vi "TP_Privileges.vi"(8 "error in (no error)":errorcluster, 10 "Privilege":T1) -> (0 "error out":errorcluster)   [LabVIEW 2012]
uses:
  TP_Privileges.ctl
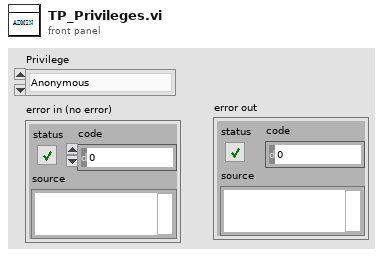
[diagram p1: front panel]
types:
  T1 = typedef "TP_Privileges.ctl" = enum16{"Anonymous", "User", "Debugger", "Developer", "Admin"}
  T2 = enum16{"Init", "GetValue", "SetValue", "Destory"}
  T3 = typedef "TP_Config.ctl" = cluster{"Info":cluster{"version":string, "date":string, "author":string, "mail":string}, "User_info":cluster{"username":string, "memery_enable":bool}, "Path":cluster{"script":string, "errlog":string}}
  T4 = typedef "TP_UI Ref.ctl" = cluster{"This VI":refnum<vi>, "String":refnum<vi>, "Test":refnum<vi>, "Quit":refnum<vi>, "SrciptList":refnum<vi>, "TRS":refnum<vi>, "Info":refnum<vi>, "Result":refnum<vi>, "menu":refnum<k9>}
  T5 = cluster{"Config":T3, "UI_Ref":T4, "Privilege":T1, "Stop":bool}
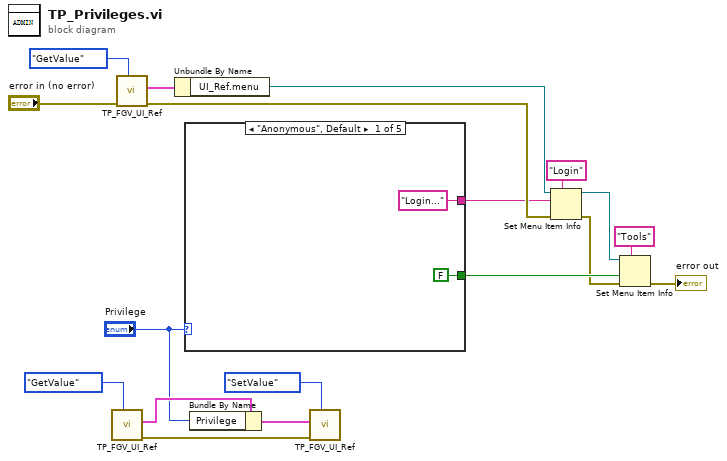
[diagram p0: block diagram]
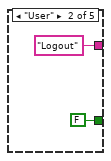
[diagram p2: hidden frame]
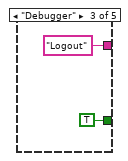
[diagram p3: hidden frame]
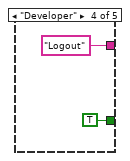
[diagram p4: hidden frame]
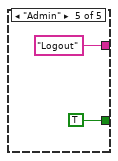
[diagram p5: hidden frame]
diagram:
  n1 = call "TP_FGV_UI_Ref.vi"("Enum"=T2."GetValue") -> ("error out"=w4:errorcluster, "Global Variants out"=w5:T5)  [unwired: 9 in]
  n2 = call "TP_FGV_UI_Ref.vi"("Enum"=T2."GetValue", "error in (no error)"="error in (no error)") -> ("error out"=w12:errorcluster, "Global Variants out"=w17:T5)  [unwired: 8 in]
  n3 = Unbundle By Name(w17) -> ("UI_Ref.menu"=w10:refnum<k9>)
  n4 = case shown="\"Anonymous\", Default" "Privilege" {
    tunnel: [FALSE ("enabled") FALSE ("enabled") TRUE ("enabled") TRUE ("enabled") TRUE ("enabled")] -> w15
    tunnel: ["Login..." ("item tag") "Logout" ("item tag") "Logout" ("item tag") "Logout" ("item tag") "Logout" ("item tag")] -> w7
    frame "Anonymous", Default {
    }
    frame "User" {
    }
    frame "Debugger" {
    }
    frame "Developer" {
    }
    frame "Admin" {
    }
  }
  n5 = Bundle By Name(cluster=w5, "Privilege"="Privilege") -> (w3:T5)
  n6 = call "TP_FGV_UI_Ref.vi"("Enum"=T2."SetValue", "error in (no error)"=w4, "Global Variants in"=w3) -> ()  [unwired: 7 in, 2 out]
  n7 = Set Menu Item Info(7:"Login" ("item tag"), 8:w12, 10:w7, 11:w10) -> (0:w11:errorcluster, 3:w9:refnum<k9>)  [unwired: 3 in]
  n8 = Set Menu Item Info(7:"Tools" ("item tag"), 8:w11, 9:w15, 11:w9) -> (0:→"error out":errorcluster)  [unwired: 3 in, 1 out]
